vi "ReadICP.vi"(8 "error in (no error)":errorcluster, 11 "DataVer3 in":refnum<class "DataVer3.lvclass">) -> (0 "error out":errorcluster, 2 "ICP":bool, 3 "DataVer3 out":refnum<class "DataVer3.lvclass">)   [LabVIEW 2013, in "DataVer3.lvclass"]
uses:
  DataVer3.lvclass
  DataVer3.lvclass/DataVer3.ctl
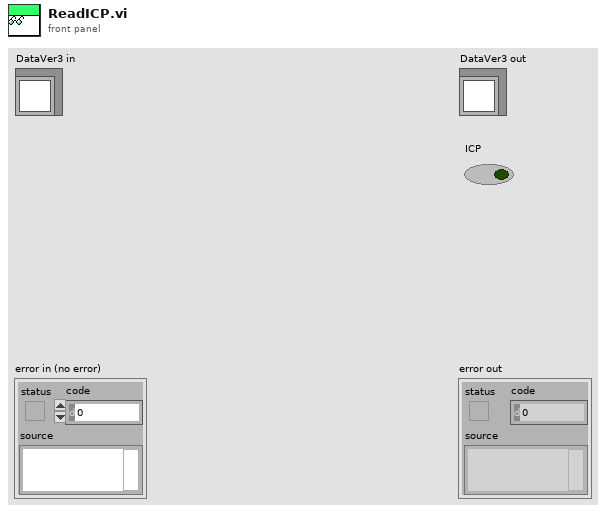
[diagram p1: front panel]
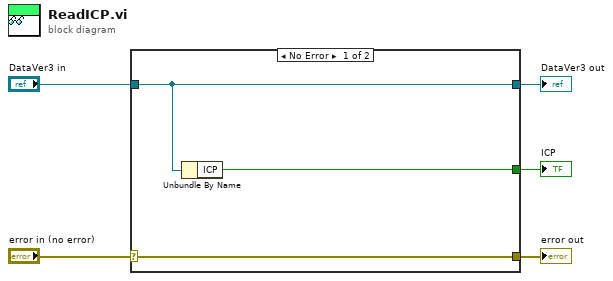
[diagram p0: block diagram]
diagram:
  n1 = case shown="No Error" "error in (no error)" {
    selector: "error in (no error)" -> [w8 w9]
    tunnel: [w8 w9] -> w4
    tunnel: [w7 w10] -> w2
    tunnel: "DataVer3 in" -> [w7 w10]
    tunnel: [w6 _] -> w1
    frame No Error {
      n2 = Unbundle By Name(w7) -> ("ICP"=w6:bool)
    }
    frame Error {
    }
  }
  "error out" <- w4
  "DataVer3 out" <- w2
  "ICP" <- w1
